vi "resultsColumnsSWrev.vi"(10 "chValuesIn":string[](array[string]), 11 "chNamesIn":string[](array[string])) -> (2 "chValuesOut":string[](array[string]), 3 "chNamesOut":string[](array[string]))   [LabVIEW 2020]
uses:
  Globals/Meas_global.vi
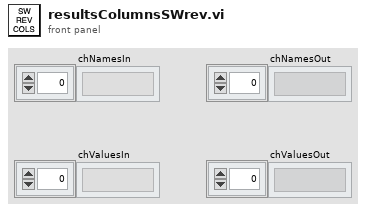
[diagram p1: front panel]
types:
  T1 = typedef "Post_Process.ctl" = enum16{"Take New Data", "Post Process Raw Data File"}
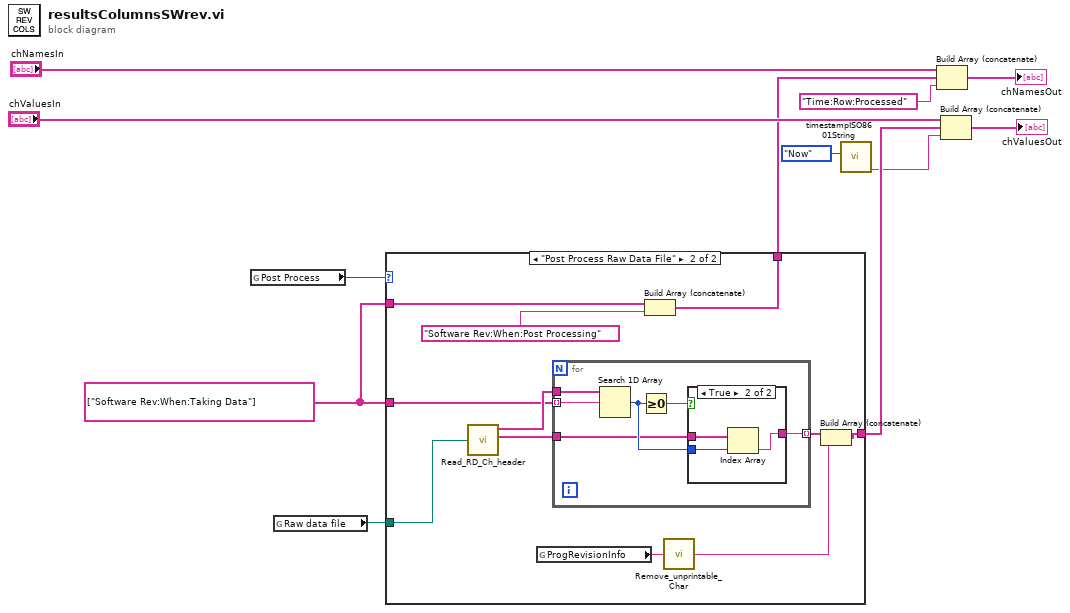
[diagram p0: block diagram]
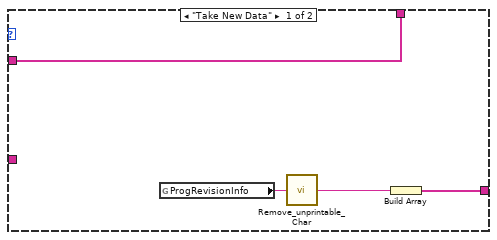
[diagram p2: hidden frame]
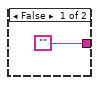
[diagram p3: hidden frame]
diagram:
  w5 = string[] ["Software Rev:When:Taking Data"] ("appended array")
  n1 = global read "Meas_global.vi" "Post Process"() -> (w8:T1)
  n2 = global read "Meas_global.vi" "Raw data file"() -> (w7:path)
  n3 = case shown="\"Post Process Raw Data File\"" w8 {
    tunnel: [w16 w18] -> w6
    tunnel: w7 -> [_ w27]
    tunnel: w5 -> [_ w24]
    tunnel: [w13 w20] -> w4
    tunnel: w5 -> [w13 w22]
    frame "Take New Data" {
      n4 = global read "Meas_global.vi" "ProgRevisionInfo"() -> (w15:string)
      n5 = call "Remove_unprintable_Char.vi"("Input String"=w15) -> ("Output String"=w14:string)
      n6 = Build Array(w14) -> (w16:string[])
    }
    frame "Post Process Raw Data File" {
      n7 = call "Read_RD_Ch_header.vi"("Raw data file"=w27) -> ("Ch Name Out"=w26:string[], "Ch Values"=w25:string[])  [unwired: 2 out]
      n8 = global read "Meas_global.vi" "ProgRevisionInfo"() -> (w21:string)
      n9 = for {
        tunnel: w26 -> [w33]
        tunnel: w25 -> [w30]
        tunnel: [w29] -> w23 mode=indexing
        tunnel: w24 -> [w28] mode=indexing
        n10 = Search 1D Array(1D array=w33, element=w28) -> (index of element=w31:i32)  [unwired: 1 out]
        n11 = Greater Or Equal To 0?(x=w31) -> (x >= 0?=w32:bool)
        n12 = case shown="True" w32 {
          tunnel: w31 -> [_ w37]
          tunnel: w30 -> [_ w36]
          tunnel: ["" w35] -> w29
          frame False {
          }
          frame True {
            n13 = Index Array(array=w36, index=w37) -> (element=w35:string)
          }
        }
      }
      n14 = Build Array (concatenate)(w22, "Software Rev:When:Post Processing" ("Input Element")) -> (w20:string[])
      n15 = call "Remove_unprintable_Char.vi"("Input String"=w21) -> ("Output String"=w17:string)
      n16 = Build Array (concatenate)(w23, w17) -> (w18:string[])
    }
  }
  n17 = call "timestampISO8601String.vi"("When?"=enum16{"Now", "Use Input"}."Now") -> ("date/timeWithSeconds"=w2:string)  [unwired: 7 in, 3 out]
  n18 = Build Array (concatenate)("chNamesIn", w4, "Time:Row:Processed" ("Input Element")) -> (→"chNamesOut":string[])
  n19 = Build Array (concatenate)("chValuesIn", w6, w2) -> (→"chValuesOut":string[])
